vi "CLD 2 Elapsed Time Express FGV Exercise.vi"(7 "Timer-Modus":T1(ring), 8 "Fehler (Eingang, kein Fehler)":errorcluster, 9 "Autom. zurücksetzen (F)":bool, 11 "Zielzeit (s)":dbl=7.0) -> (0 "Fehler (Ausgang)":errorcluster, 2 "Verstrichene Zeit (s)":dbl, 3 "Zeit ist verstrichen":bool)   [LabVIEW 2014]
doc: "Functional global: Elapsed Time, getter and setter dependent on \"timer mode\" enum. CLD-Übung 2"
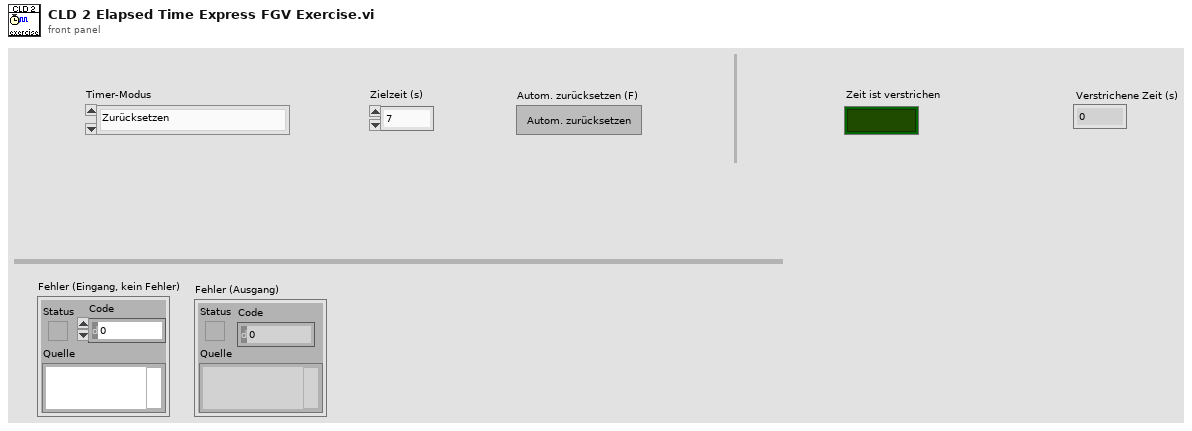
[diagram p1: front panel]
types:
  T1 = enum16{"Zurücksetzen", "Status abfragen", "Autom. Zurücksetzen festlegen"}
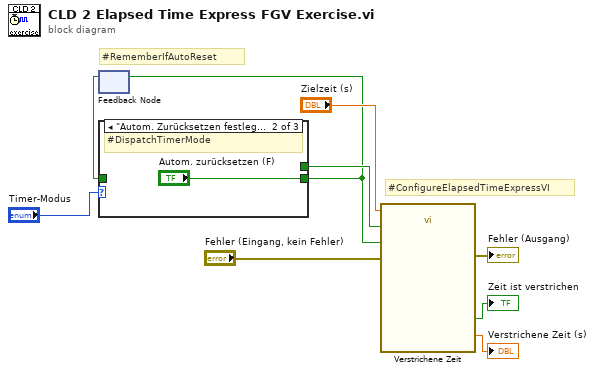
[diagram p0: block diagram]
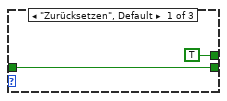
[diagram p2: hidden frame]
diagram:
  # "#ConfigureElapsedTimeExpressVI"
  # "#RememberIfAutoReset"
  n1 = feedback #1 ("Rückkopplungsknoten")() -> (w2:bool)  [unwired: 1 in]
  n2 = case shown="\"Autom. Zurücksetzen festlegen\"" "Timer-Modus" {
    tunnel: [TRUE _ _] -> w3
    tunnel: [w10 "Autom. zurücksetzen (F)" w13] -> w1
    tunnel: w2 -> [w10 _ w13]
    frame "Zurücksetzen", Default {
    }
    frame "Autom. Zurücksetzen festlegen" {
      # "#DispatchTimerMode"
    }
    frame "Status abfragen" {
    }
  }
  n3 = feedback-in #1(w1) -> ()
  n4 = call "Verstrichene Zeit"("Time Target (s)"="Zielzeit (s)", "Reset"=w3, "Auto Reset"=w1, "error in (no error)"="Fehler (Eingang, kein Fehler)") -> ("Elapsed Time (s)"=→"Verstrichene Zeit (s)":dbl, "Time has Elapsed"=→"Zeit ist verstrichen":bool, "error out"=→"Fehler (Ausgang)":errorcluster)  [unwired: 8 in, 5 out]
